vi "Retriggerable Analog Input (STC3).vi"() -> ()   [LabVIEW 2009]
uses:
  <vilib>/DAQmx/configure/trigger.llb/DAQmx Start Trigger (Digital Edge).vi
  <vilib>/DAQmx/configure/timing.llb/DAQmx Timing (Sample Clock).vi
  <vilib>/DAQmx/create/channels.llb/DAQmx Create Channel (AI-Voltage-Basic).vi
  <vilib>/DAQmx/read.llb/DAQmx Read (Analog 1D DBL 1Chan NSamp).vi
  Program Files/National Instruments/LabVIEW 2009/resource/objmgr/daqmx.rc
panel:
  in  "samples per channel":i32=1000
  out "data":dbl[](graph)=[0.11633395532614343, 2.322477792337649, 2.49304052741351, 2.4512898694732237, 0.7765741109067276, -1.6028776767751645, -2.866070770695397, -2.8212456872470555, -1.0924868869830124, 1.3269366026043294]
  in  "stop":bool
  in  "rate":dbl=1000.0 format="%0.2f"
  in  "analog input channels":tag="Dev1/ai2"
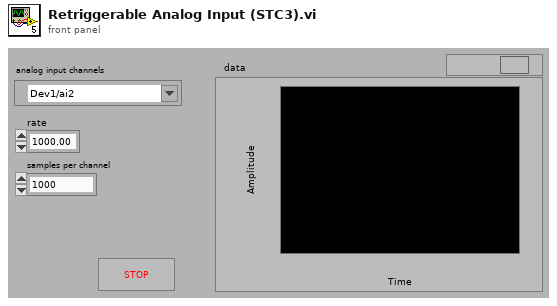
[diagram p1: front panel]
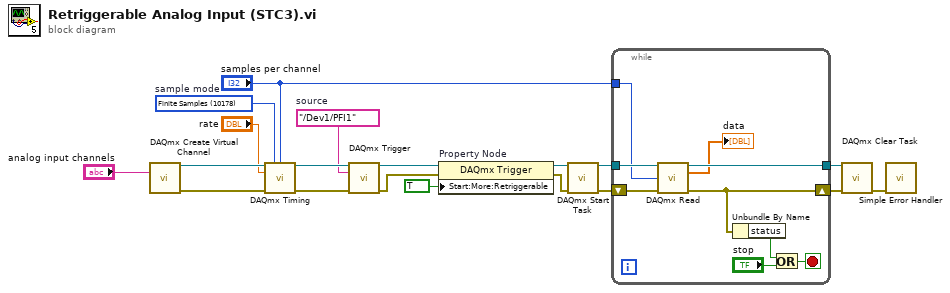
[diagram p0: block diagram]
diagram:
  w12 = tag "/Dev1/PFI1"  # source
  w16 = 10178 items=["Finite Samples"=10178, "Continuous Samples"=10123, "Hardware Timed Single Point"=12522]  # sample mode
  n1 = call-poly <vilib>:"DAQmx Create Virtual Channel.vi"("physical channels"="analog input channels") -> ("task out"=w19:refnum<k21>, "error out"=w18:errorcluster)  [unwired: 13 in]
  n2 = call-poly <vilib>:"DAQmx Timing.vi"("task/channels in"=w19, "sample mode"=w16, "samples per channel"="samples per channel", "rate"="rate", "error in"=w18) -> ("task out"=w14:refnum<k21>, "error out"=w13:errorcluster)  [unwired: 9 in]
  n3 = call-poly <vilib>:"DAQmx Trigger.vi"("task/channels in"=w14, "source"=w12, "error in"=w13) -> ("task out"=w11:refnum<k21>, "error out"=w9:errorcluster)  [unwired: 11 in]
  n4 = property on="Property Node" class="DAQmx Trigger"(reference=w11, error in=w9, "Start:More:Retriggerable"=TRUE ("Start.Retriggerable")) -> (reference out=w10:refnum<k21>, error out=w8:errorcluster)
  n5 = call <vilib>:"DAQmx Start Task.vi"("task/channels in"=w10, "error in"=w8) -> ("task out"=w6:refnum<k21>, "error out"=w5:errorcluster)  [unwired: 12 in]
  n6 = while {
    tunnel: w6 -> [w28]
    tunnel: [w26] -> w3
    tunnel: "samples per channel" -> [w20]
    shift-right: [w23] -> w2
    shift-left: w5 -> [w27]
    stop <- w22 stop-if-true
    n7 = call-poly <vilib>:"DAQmx Read.vi"("task/channels in"=w28, "number of samples per channel"=w20, "error in"=w27) -> ("task out"=w26:refnum<k21>, "data"=→"data":dbl[], "error out"=w23:errorcluster)  [unwired: 10 in]
    n8 = Unbundle By Name "Unbundle By Name"(w23) -> ("status"=w25:bool)
    n9 = Or(x=w25, y="stop") -> (x .or. y?=w22:bool)
  }
  n10 = call <vilib>:"DAQmx Clear Task.vi"("task in"=w3, "error in"=w2) -> ("error out"=w4:errorcluster)  [unwired: 13 in]
  n11 = call <vilib>:"Simple Error Handler.vi"("error in (no error)"=w4) -> ()  [unwired: 4 in, 5 out]
